vi "rwr_Stop Measurement.vi"(4 "Show in Debugger?":bool=TRUE, 6 "Message Priority":T1=enum."Normal", 7 "Caller in":refnum<class "Worker.lvclass">, 8 "error in":errorcluster, 9 "timeout (ms)":i32=5000, 10 "Data in":T3, 11 "DMM HAL in":refnum<class "DMM HAL.lvclass">) -> (0 "error out":errorcluster, 2 "Reply Data out":T2, 3 "dup DMM HAL out":refnum<class "DMM HAL.lvclass">)   [LabVIEW 2020, in "DMM HAL.lvclass"]
doc: "This VI sends a <b>Public API Request with Reply</b> message to an MHL case of the Worker that owns this VI. This VI will wait until it receives a <b>Reply</b> message back from the Worker that owns this VI. If the wait time exceeds <b>timeout (ms)</b>, an error will be returned.\n---\nStop the DMM measurement."
uses:
  DMM HAL.lvclass
  <vilib>/addons/_Workers/Library/Classes/Worker/Worker.lvclass
  rwr_Stop Measurement.ctl
  rwr_Stop Measurement Reply.ctl
  <vilib>/addons/_Workers/Library/Classes/Message/Priority.ctl
  <vilib>/addons/_Workers/Library/Classes/Message/Message.lvclass
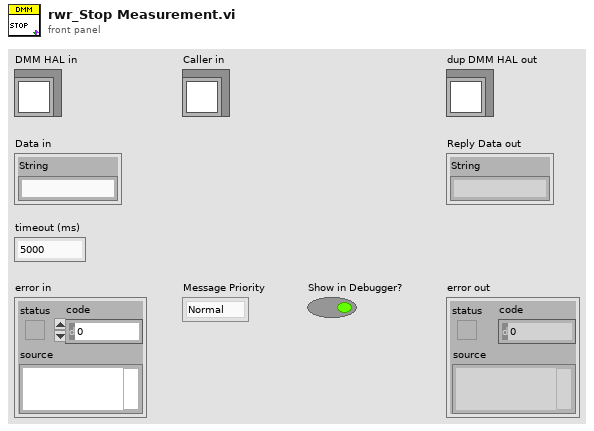
[diagram p1: front panel]
types:
  T1 = typedef "Workers.lvlib/Message.lvclass/Priority.ctl" = enum16{"Low", "Normal", "High"}
  T2 = typedef "DMM HAL.lvclass/rwr_Stop Measurement Reply.ctl" = cluster{"String":string}
  T3 = typedef "DMM HAL.lvclass/rwr_Stop Measurement.ctl" = cluster{"String":string}
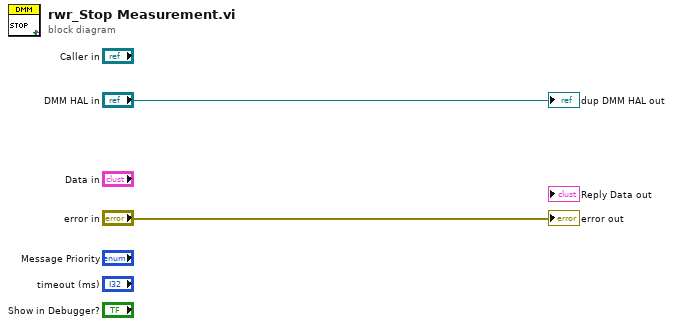
[diagram p0: block diagram]
diagram:
  "error out" <- "error in"
  "dup DMM HAL out" <- "DMM HAL in"
